vi "Get Local UTC Offset.vi"(10 "UTC? (F)":bool) -> (1 "UTC Offset String":string, 2 "UTC Offset":T1=enum."UTC+00:00")   [LabVIEW 2021]
uses:
  UTC Offsets -- enum.ctl
  <vilib>/Utility/miscctls.llb/LVDateTimeRec.ctl
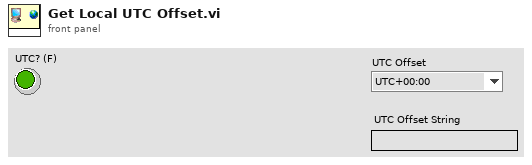
[diagram p1: front panel]
types:
  T1 = typedef "UTC Offsets -- enum.ctl" = enum16{"UTC-12:00", "UTC-11:00", "UTC-10:00", "UTC-09:30", "UTC-09:00", "UTC-08:00", "UTC-07:00", "UTC-06:00", "UTC-05:00", "UTC-04:00", "UTC-03:30", "UTC-03:00", "UTC-02:00", "UTC-01:00", "UTC-00:00", "UTC+00:00", "UTC+01:00", "UTC+02:00", "UTC+03:00", "UTC+03:30", "UTC+04:00", "UTC+04:30", "UTC+05:00", "UTC+05:30", "UTC+05:45", "UTC+06:00", "UTC+06:30", "UTC+07:00", "UTC+08:00", "UTC+08:45", "UTC+09:00", "UTC+09:30", "UTC+10:00", "UTC+10:30", "UTC+11:00", "UTC+12:00", "UTC+12:45", "UTC+13:00", "UTC+14:00"}
  T2 = typedef "LVDateTimeRec.ctl" = cluster{"fractional second":dbl, "second":i32, "minute":i32, "hour":i32, "day of month":i32, "month":i32, "year":i32, "day of week":i32, "day of year":i32, "DST":i32}
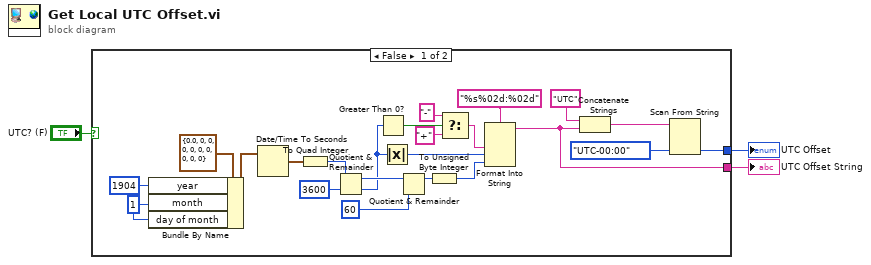
[diagram p0: block diagram]
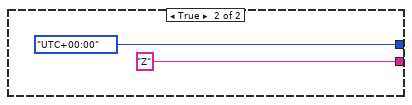
[diagram p2: hidden frame]
diagram:
  n1 = case shown="False" "UTC? (F)" {
    tunnel: [w22 UTC_Offsets_--_enum."UTC+00:00" ("UTC Time Offset")] -> w3
    tunnel: [w9 "Z"] -> w2
    frame False {
      w8 = 1 ("month")
      n2 = Bundle By Name(cluster=T2 {"fractional second"=0.0, "second"=0, "minute"=0, "hour"=0, "day of month"=0, "month"=0, "year"=0, "day of week"=0, "day of year"=0, "DST"=0} ("date time rec"), "year"=1904, "month"=w8, "day of month"=w8) -> (w6:T2)
      n3 = Date/Time To Seconds(2:w6) -> (0:w4:timestamp)  [unwired: 1 in]
      n4 = To Quad Integer(1:w4) -> (0:w14:i64)
      n5 = Quotient & Remainder(x=w14, y=i64 3600) -> (x-y*floor(x/y)=w17:i64, floor(x/y)=w15:i64)
      n6 = Greater Than 0?(x=w15) -> (x > 0?=w21:bool)
      n7 = Absolute Value(x=w15) -> (abs(x)=w18:i64)
      n8 = Quotient & Remainder(x=w17, y=i64 60) -> (x-y*floor(x/y)=w25:i64)  [unwired: 1 out]
      n9 = To Unsigned Byte Integer(number=w25) -> (unsigned 8bit integer=w24:u8)
      n10 = Select(t="-" ("format string"), s=w21, f="+" ("format string")) -> (s? t:f=w12:string)
      n11 = Format Into String(format string="%s%02d:%02d", w12, w18, w24) -> (resulting string=w9:string)  [unwired: 2 in, 1 out]
      n12 = Concatenate Strings("UTC" ("format string"), w9) -> (w11:string)
      n13 = Scan From String(input string=w11, default 1=UTC_Offsets_--_enum."UTC-00:00" ("UTC Time Offset")) -> (output 1=w22:T1)  [unwired: 3 in, 3 out]
    }
    frame True {
    }
  }
  "UTC Offset" <- w3
  "UTC Offset String" <- w2
